vi "Convert Global Velocity to Steering Frame.vi"(10 "steering frame angle (rad)":dbl, 11 "global velocity":dbl[](array[numeric])=[0.0, 0.0, 0.0]) -> (3 "steering frame velocity":dbl[](array[numeric]))   [LabVIEW 2017, in "NI_Robotics_Steering Frame.lvclass"]
uses:
  <vilib>/robotics/Steering/Steering Frame/NI_Robotics_Steering Frame.lvclass
  <vilib>/Analysis/coordinate.llb/2D Cartesian Coordinate Rotation (Scalar).vi
  <vilib>/Analysis/NI_AALPro.lvlib
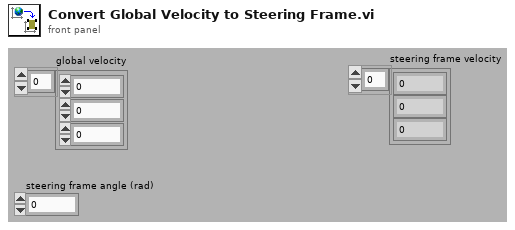
[diagram p1: front panel]
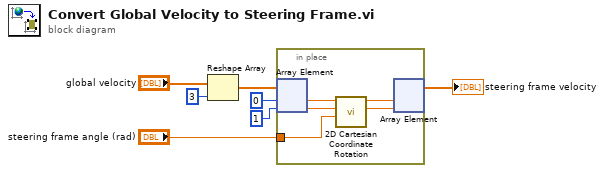
[diagram p0: block diagram]
diagram:
  n1 = Reshape Array("global velocity", 3 ("dimension size")) -> (w5:dbl[])
  n2 = in-place {
    in-place-border: "steering frame angle (rad)" -> [w8]
    n3 = in-place-array #1(w5, 0, 1) -> (w12:dbl, w11:dbl)
    n4 = call-poly <vilib>:"2D Cartesian Coordinate Rotation.vi"("theta"=w8, "y"=w11, "x"=w12) -> ("y out"=w9:dbl, "x out"=w10:dbl)  [unwired: 6 in, 1 out]
    n5 = in-place-array #1(w10, w9) -> (→"steering frame velocity":dbl[])  [unwired: 2 out]
  }
